vi "save scale.vi"(5 "Folder":T1, 7 "error in (no error)":errorcluster, 10 "Index":u32) -> (0 "error":errorcluster)   [LabVIEW 2015]
uses:
  Process Controller 3.0/Calibration and Function folders.ctl
  DAQ configuration/Sensor buffer command.ctl
panel:
  in  "calibration file path":enum16{""}(ring)
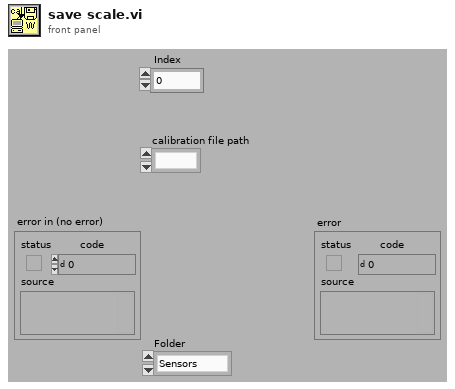
[diagram p1: front panel]
types:
  T1 = typedef "Calibration and Function folders.ctl" = enum16{"Sensors", "Functions", "Config File", "PublicAppFolder", "New ini File", "Set Config File", "Delete ini File"}
  T2 = typedef "Sensor buffer command.ctl" = enum16{"read average", "read recent", "read all", "write", "set buffer size", "Read channel config", "Write channel config", "clear"}
  T3 = enum16{"open", "open or create", "create or replace", "create", "open (read only)"}
  T4 = typedef "Channel config.ctl" = cluster{"Channel Indices":T5[], "AI Max voltage":dbl[], "Calibration matrix":T6}
  T5 = typedef "channel identifier.ctl" = u16
  T6 = typedef "calib array.ctl" = T7[]
  T7 = typedef "conversion.ctl" = cluster{"conversion matrix":sgl[][], "units":string, "name":string, "scale type":T8, "offset (volts)":dbl, "second channel":i8, "correspondence table":T9, "offset (physical units)":dbl, "pH scale":T10, "D.O.":T11, "Photometer data":T12}
  T8 = typedef "scale type.ctl" = enum16{"Volts", "Polynomial", "Correspondence Table", "pH", "Dissolved Oxygen", "Quadratic", "Photometer"}
  T9 = typedef "correspondence table.ctl" = cluster{"physical units":dbl, "volts":dbl}[]
  T10 = typedef "pH scale.ctl" = cluster{"Buffers":cluster{"Buffer":dbl, "Calibrated":bool, "V/T":dbl}[], "Temperature":dbl}
  T11 = typedef "DO scale.ctl" = cluster{"Temperature":dbl, "K":dbl, "barometric pressure":dbl}
  T12 = typedef "Photometer calibration data.ctl" = cluster{"Dark Voltage":dbl, "Blank Voltage":dbl, "Standards":cluster{"Concentration":dbl, "Voltage":dbl}[]}
  T13 = enum16{"open", "replace", "create", "open or create", "replace or create", "replace or create with confirmation"}
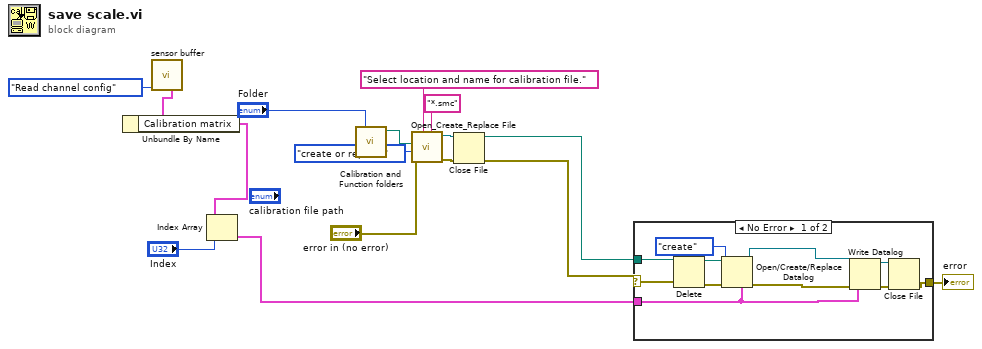
[diagram p0: block diagram]
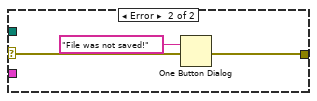
[diagram p2: hidden frame]
diagram:
  n1 = call "sensor buffer.vi"("command"=Sensor_buffer_command."Read channel config") -> ("Channel Config out"=w5:T4)  [unwired: 6 in, 4 out]
  n2 = Unbundle By Name(w5) -> ("Calibration matrix"=w4:T6)
  n3 = Index Array(array=w4, index="Index") -> (element=w7:T7)
  n4 = call "Calibration and Function folders.vi"("Folder"="Folder") -> ("Selected Folder"=w3:path)  [unwired: 9 in, 1 out]
  n5 = call <vilib>:"Open_Create_Replace File.vi"("pattern"="*.smc", "prompt"="Select location and name for calibration file.", "error in (no error)"="error in (no error)", "function (open:0)"=T3."create or replace", "start path  (Not A Path)"=w3) -> ("error out"=w14:errorcluster, "refnum"=w13:refnum<file>)  [unwired: 3 in, 2 out]
  n6 = Close File(refnum=w13, error in=w14) -> (path=w8:path, error out=w10:errorcluster)
  n7 = case shown="No Error" w10 {
    selector: w10 -> [w21 w28]
    tunnel: w8 -> [w19 _]
    tunnel: w7 -> [w24 _]
    tunnel: [w25 w28] -> w11
    frame No Error {
      n8 = Delete(path (use dialog)=w19, error in=w21) -> (deleted path=w18:path, error out=w20:errorcluster)  [unwired: 3 in, 1 out]
      n9 = Open/Create/Replace Datalog(5:w24, 8:w20, 10:T13."create" ("operation (0:open)"), 11:w18) -> (0:w22:errorcluster, 3:w23:refnum<k1>)  [unwired: 2 in, 1 out]
      n10 = Write Datalog(4:w22, 6:w24, 7:w23) -> (0:w27:errorcluster, 3:w26:refnum<k1>)
      n11 = Close File(refnum=w26, error in=w27) -> (error out=w25:errorcluster)  [unwired: 1 out]
    }
    frame Error {
      n12 = One Button Dialog(message="File was not saved!") -> ()  [unwired: 1 in, 1 out]
    }
  }
  "error" <- w11
